vi "Resolve To Pins from Group.vi"(10 "group mappings":T1, 11 "pin or relay or its group names":string[](array[string])) -> (3 "resolved pin or relay names":string[](array[string]))   [LabVIEW 2020, in "MeasurementLink Session Management V1.lvlib" / "Session Reservation.lvclass"]
doc: "If a given pin or relay name is a group name then resolve them to pins and append them."
uses:
  Session Reservation.lvclass
  Group Mapping.ctl
  41dee1a7-95a6-4112-bccc-97afb29f1749.vi
panel:
  # "Outputs"
  # "Inputs"
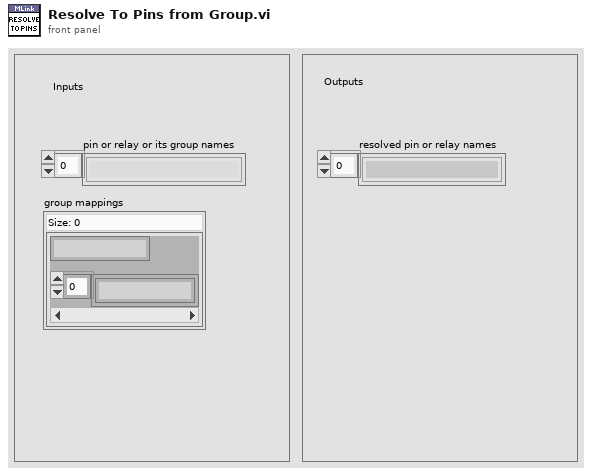
[diagram p1: front panel]
types:
  T1 = typedef "MeasurementLink Session Management V1.lvlib/Session Reservation.lvclass/Group Mapping.ctl" = map{string, string[]}
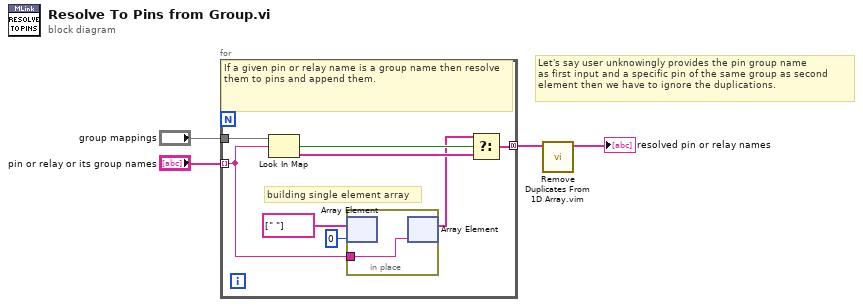
[diagram p0: block diagram]
diagram:
  # "Let's say user unknowingly provides the pin group name \nas first input and a specific pin of the same group as second\nelement then we have to ignore the duplications."
  n1 = for {
    tunnel: "pin or relay or its group names" -> [w6] mode=indexing
    tunnel: "group mappings" -> [w12]
    tunnel: [w10] -> w2 mode=concatenating
    # "building single element array"
    # "If a given pin or relay name is a group name then resolve them to pins and append them."
    n2 = Look In Map(map=w12, key=w6) -> (key not found?=w11:bool, value=w9:string[])  [unwired: 1 in]
    n3 = in-place {
      in-place-border: w6 -> [w13]
      n4 = in-place-array #1(string[] [" "] ("appended array"), 0) -> ()  [unwired: 1 out]
      n5 = in-place-array #1(w13) -> (w5:string[])  [unwired: 1 out]
    }
    n6 = Select(t=w5, s=w11, f=w9) -> (s? t:f=w10:string[])
  }
  n7 = call "Remove Duplicates From 1D Array.vim"("array"=w2) -> ("array with duplicates removed"=→"resolved pin or relay names":string[])  [unwired: 10 in]
